vi "SetAllCamPara.vi"(1 "曝光时间1?":bool, 2 "ImgProcessOutput out":T1) -> (0 "Result":bool)   [LabVIEW 2014]
uses:
  ImgProcessOutput.ctl
  <vilib>/userdefined/High Color/IMAQdx.ctl
  Controls/MsgAction.ctl
panel:
  out "数值":u32
  # "%"
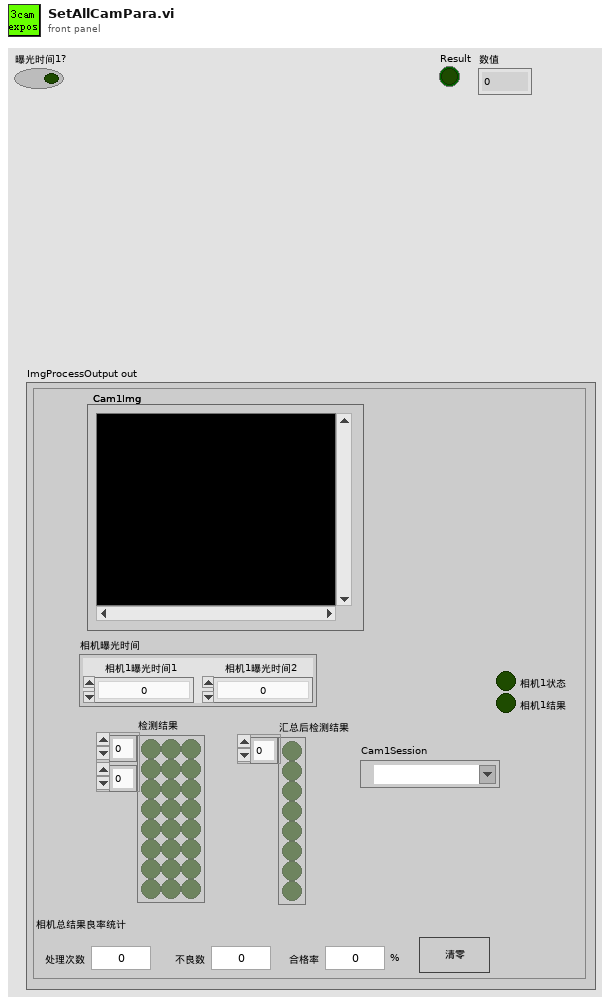
[diagram p1: front panel]
types:
  T1 = typedef "ImgProcessOutput.ctl" = cluster{"Cam1Img":T2, "Cam1Session":T3, "相机1状态":bool, "相机1结果":bool, "相机曝光时间":cluster{"相机1曝光时间1":i32, "相机1曝光时间2":i32}, "检测结果":bool[][], "汇总后检测结果":bool[], "相机总结果良率统计":T4}
  T2 = typedef "IMAQ Image.ctl" = refnum<image>
  T3 = typedef "IMAQdx.ctl" = refnum<k21>
  T4 = typedef "ProductNum.ctl" = cluster{"处理次数":u64, "不良数":u64, "合格率":dbl, "清零":bool}
  T5 = typedef "MsgAction.ctl" = enum16{"初始化", "添加消息", "区分结果添加消息", "清空消息", "获取消息"}
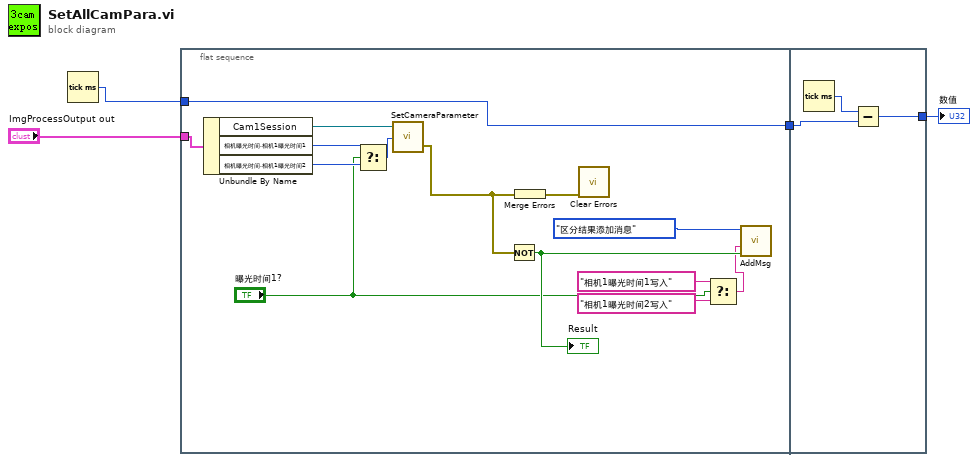
[diagram p0: block diagram]
diagram:
  n1 = Tick Count (ms)() -> (millisecond timer value=w3:u32)
  n2 = flat-sequence {
    tunnel: "ImgProcessOutput out" -> [w17]
    tunnel: w3 -> [w9]
    tunnel: [w9] -> w2
    tunnel: w2 -> [w20]
    tunnel: [w19] -> w1
    frame #0 {
      n3 = Unbundle By Name(w17) -> ("Cam1Session"=w16:T3, "相机曝光时间.相机1曝光时间1"=w8:i32, "相机曝光时间.相机1曝光时间2"=w7:i32)
      n4 = Select(t=w8, s="曝光时间1?", f=w7) -> (s? t:f=w6:i32)
      n5 = call "SetCameraParameter.vi"("Exposure time"=w6, "Session In"=w16) -> ("error out"=w15:errorcluster)  [unwired: 1 in, 1 out]
      n6 = Not(x=w15) -> (.not. x?=w13:bool)
      "Result" <- w13
      n7 = Merge Errors(w15) -> (w18:errorcluster)
      n8 = call <vilib>:"Clear Errors.vi"("error in (no error)"=w18) -> ()  [unwired: 5 in, 2 out]
      n9 = Select(t="相机1曝光时间1写入" ("添加消息"), s="曝光时间1?", f="相机1曝光时间2写入" ("添加消息")) -> (s? t:f=w10:string)
      n10 = call "AddMsg.vi"("Result"=w13, "添加消息"=w10, "消息Action"=MsgAction."区分结果添加消息") -> ()  [unwired: 1 in, 1 out]
    }
    frame #1 {
      n11 = Tick Count (ms)() -> (millisecond timer value=w21:u32)
      n12 = Subtract(x=w21, y=w20) -> (x-y=w19:u32)
    }
  }
  "数值" <- w1
